vi "UI - Memory.vi"(5 "Term (Methods)":string="Methods", 7 "Msg Chain":string, 8 "error in (no error)":errorcluster {"code" format="Error %.0f"}, 10 "UI Docs":refnum<class "GUI Documentation.lvclass">[](array[class]), 11 "VIDoc Printer - Confluence In":refnum<class "VIDoc Printer - Confluence.lvclass">) -> (0 "error out":errorcluster {"code" format="Error %.0f"}, 3 "VIDoc Printer - Confluence Out":refnum<class "VIDoc Printer - Confluence.lvclass">)   [LabVIEW 2023, in "VIDoc Printer - Confluence.lvlib" / "VIDoc Printer - Confluence.lvclass"]
doc: "Generates the specific UI Type Memory section."
uses:
  VIDoc Printer - Confluence.lvclass
  VIDoc Printer - Confluence.lvclass/VIDoc Printer - Confluence.ctl
  Confluence Formatting/Confluence Formatting.lvlib
  Confluence Formatting/Types/Format Combo Box.ctl
  Parsing/GUI Documentation/GUI Documentation.lvclass
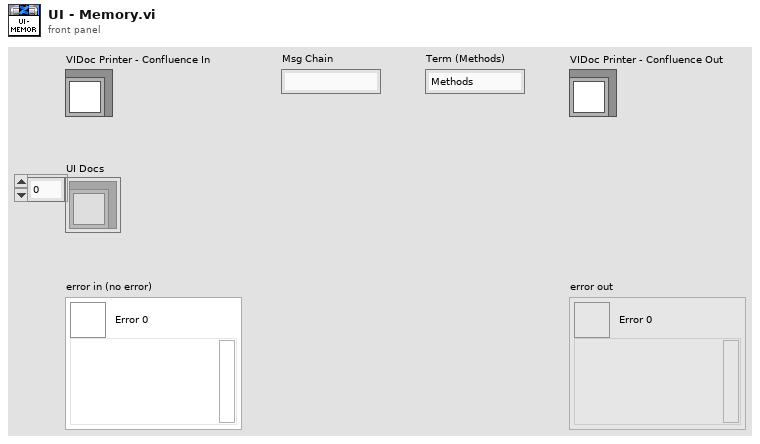
[diagram p1: front panel]
types:
  T1 = typedef "Confluence Formatting.lvlib/Format Combo Box.ctl" = string
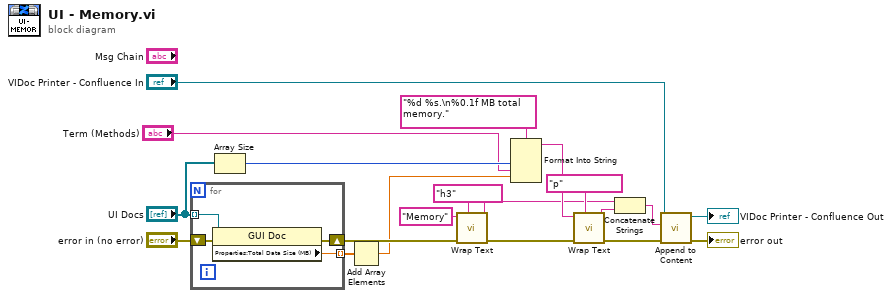
[diagram p0: block diagram]
diagram:
  n1 = for {
    tunnel: "UI Docs" -> [w23] mode=indexing
    tunnel: [w22] -> w12 mode=indexing
    shift-right: [w21] -> w11
    shift-left: "error in (no error)" -> [w24]
    n2 = property class="GUI Doc"(reference=w23, error in=w24) -> (error out=w21:errorcluster, "Properties:Total Data Size (MB)"=w22:dbl)  [unwired: 1 out]
  }
  n3 = Array Size(array="UI Docs") -> (size(s)=w3:i32)
  n4 = Add Array Elements(numeric array=w12) -> (sum=w2:dbl)
  n5 = call "Wrap Text.vi"("Formatting"=T1 "h3", "Error in"=w11, "String"="Memory") -> ("Error out"=w18:errorcluster, "Wrapped String"=w6:string)  [unwired: 7 in]
  n6 = Format Into String(format string="%d %s.\n%0.1f MB total memory.", w3, "Term (Methods)", w2) -> (resulting string=w8:string)  [unwired: 2 in, 1 out]
  n7 = call "Wrap Text.vi"("Formatting"=T1 "p", "Error in"=w18, "String"=w8) -> ("Error out"=w17:errorcluster, "Wrapped String"=w5:string)  [unwired: 7 in]
  n8 = Concatenate Strings(w6, w5) -> (w4:string)
  n9 = call "Append to Content.vi"("error in (no error)"=w17, "Content"=w4, "VIDoc Printer - Confluence In"="VIDoc Printer - Confluence In") -> ("error out"=→"error out":errorcluster, "VIDoc Printer - Confluence Out"=→"VIDoc Printer - Confluence Out":refnum<class "VIDoc Printer - Confluence.lvclass">)  [unwired: 7 in]
